vi "XLP80_EIP_End.vi"(8 "err in":errorcluster caption="error") -> (0 "err out":errorcluster caption="error")   [LabVIEW 2021]
uses:
  XLP80_General_Libs/Kirschenhofer_Libs/KH EthernetIP 17.19/KH_EthernetIP_Globals.vi
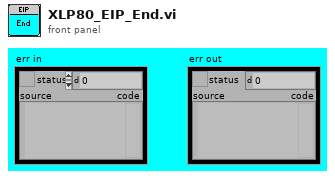
[diagram p1: front panel]
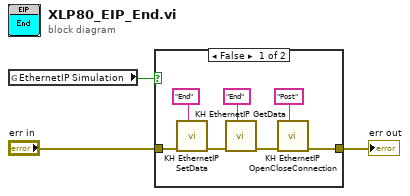
[diagram p0: block diagram]
diagram:
  n1 = global read "KH_EthernetIP_Globals.vi" "EthernetIP Simulation"() -> (w1:bool)
  n2 = case shown="False" w1 {
    tunnel: "err in" -> [w7 w11]
    tunnel: [w4 w11] -> w2
    frame False {
      n3 = call "KH EthernetIP SetData.vi"("Function"="End", "error in"=w7) -> ("error out"=w6:errorcluster)  [unwired: 7 in, 2 out]
      n4 = call "KH EthernetIP GetData.vi"("Function"="End", "error in"=w6) -> ("error out"=w5:errorcluster)  [unwired: 8 in, 1 out]
      n5 = call "KH EthernetIP OpenCloseConnection.vi"("Function"="Post", "error in"=w5) -> ("error out"=w4:errorcluster)  [unwired: 9 in]
    }
    frame True {
    }
  }
  "err out" <- w2
